vi "Model--Get Active Name.vi"(8 "error in":errorcluster, 11 "Selector in":refnum<class "Selector.lvclass">) -> (0 "error out":errorcluster, 2 "Name":string, 3 "Selector out":refnum<class "Selector.lvclass">)   [LabVIEW 2019, in "Selector.lvclass"]
uses:
  Selector.lvclass
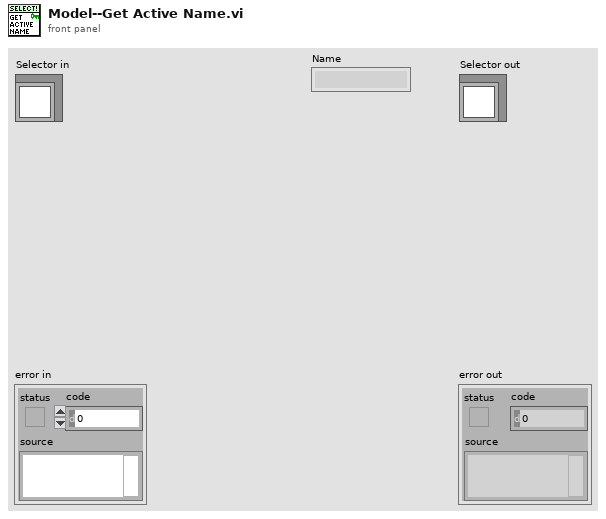
[diagram p1: front panel]
types:
  T1 = typedef "Selector.lvclass/Item.ctl" = cluster{"Name":string, "Group":string, "Enabled":bool}
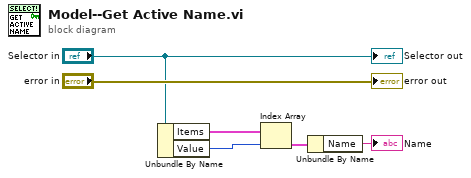
[diagram p0: block diagram]
diagram:
  n1 = Unbundle By Name("Selector in") -> ("Items"=w4:T1[], "Value"=w3:i32)
  n2 = Index Array(array=w4, index=w3) -> (element=w2:T1)
  n3 = Unbundle By Name(w2) -> ("Name"=→"Name":string)
  "error out" <- "error in"
  "Selector out" <- "Selector in"
